vi "Write Sense_Point.vi"(8 "error in":errorcluster, 10 "Sense Point":T1, 11 "69X_79X in":refnum<class "79XRP.lvclass">) -> (0 "error out":errorcluster, 3 "69X_79X out":refnum<class "79XRP.lvclass">)   [LabVIEW 2019, in "79XRP.lvlib" / "79XRP.lvclass"]
uses:
  Library/79XRP.lvclass
  C:/Users/Public/Documents/Development/builds/Instruments/PowerSupply.lvlibp/Library/PowerSupply.lvclass
  C:/Users/Public/Documents/Development/builds/Engine/Monitored Actor.lvlibp/Monitored Actor/Monitored Actor/Monitored Actor.lvclass
  builds/Instruments/PowerSupply.lvlibp/Custom Controls/Sense Point.ctl
  builds/Engine/Monitored Actor.lvlibp/Monitored Actor/Monitored Actor/Read Actor Label.vi
  <vilib>/ErrorRing/Error Ring.xnode
  builds/Instruments/PowerSupply.lvlibp/Library/PowerSupply.lvclass
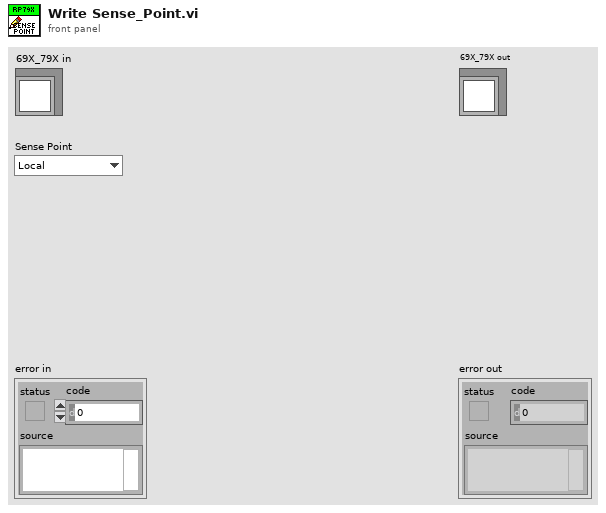
[diagram p1: front panel]
types:
  T1 = typedef "PowerSupply.lvlibp/PowerSupply.lvclass/Sense Point.ctl" = enum16{"Local", "Remote"}
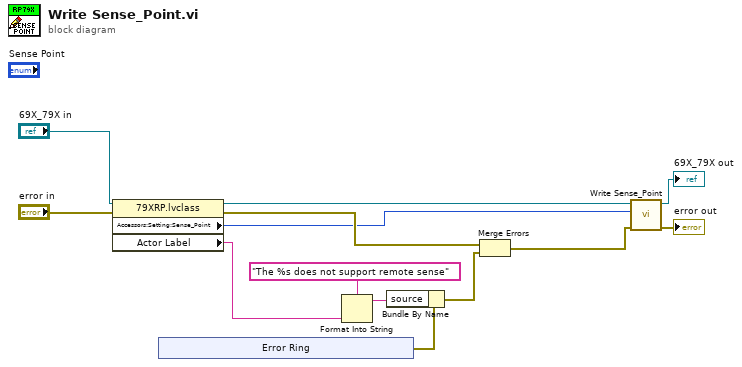
[diagram p0: block diagram]
diagram:
  n1 = property class="79XRP.lvclass"(reference="69X_79X in", error in="error in") -> (reference out=w2:refnum<class "79XRP.lvclass">, error out=w11:errorcluster, "Accessors:Setting:Sense_Point"=w3:T1, "Actor Label"=w7:string)
  n2 = xnode "Error Ring"() -> ("error out"=w10:errorcluster)
  n3 = Format Into String(format string="The %s does not support remote sense", w7) -> (resulting string=w9:string)  [unwired: 2 in, 1 out]
  n4 = Bundle By Name(cluster=w10, "source"=w9) -> (w8:errorcluster)
  n5 = Merge Errors(w11, w8) -> (w1:errorcluster)
  n6 = call-parent "Write Sense_Point.vi"("error in"=w1, "Sense Point"=w3, "PowerSupply in"=w2) -> ("error out"=→"error out":errorcluster, "PowerSupply out"=→"69X_79X out":refnum<class "79XRP.lvclass">)  [unwired: 7 in]
